vi "Read.vi"(8 "error in":errorcluster, 11 "TPCANHandle in":T2=81 items=["PCAN_NONEBUS"=0, "PCAN_USBBUS1"=81, "PCAN_USBBUS2"=82, "PCAN_USBBUS3"=83, "PCAN_USBBUS4"=84, "PCAN_USBBUS5"=85, "PCAN_USBBUS6"=86, "PCAN_USBBUS7"=87, "PCAN_USBBUS8"=88, "PCAN_USBBUS9"=1289, "PCAN_USBBUS10"=1290, "PCAN_USBBUS11"=1291, "PCAN_USBBUS12"=1292, "PCAN_USBBUS13"=1293, "PCAN_USBBUS14"=1294, "PCAN_USBBUS15"=1295, "PCAN_USBBUS16"=1296]) -> (0 "error out":errorcluster, 1 "Time Stamp":timestamp format="%<%x %.3X>T", 2 "PCAN Message":T3 {"DATA"."7" format="%.0x"; "DATA"."6" format="%.0x"; "DATA"."5" format="%.0x"; "DATA"."4" format="%.0x"; "DATA"."3" format="%.0x"; "DATA"."2" format="%.0x"; "DATA"."1" format="%.0x"; "DATA"."0" format="%.0x"; "MSGTYPE" items=["STANDARD"=0, "RTR"=1, "EXTENDED"=2, "FD"=4, "BRS"=8, "ESI"=16, "ECHO"=32, "ERRFRAME"=64, "STATUS"=128]}, 3 "TPCANHandle out":T2=81 items=["PCAN_NONEBUS"=0, "PCAN_USBBUS1"=81, "PCAN_USBBUS2"=82, "PCAN_USBBUS3"=83, "PCAN_USBBUS4"=84, "PCAN_USBBUS5"=85, "PCAN_USBBUS6"=86, "PCAN_USBBUS7"=87, "PCAN_USBBUS8"=88, "PCAN_USBBUS9"=1289, "PCAN_USBBUS10"=1290, "PCAN_USBBUS11"=1291, "PCAN_USBBUS12"=1292, "PCAN_USBBUS13"=1293, "PCAN_USBBUS14"=1294, "PCAN_USBBUS15"=1295, "PCAN_USBBUS16"=1296], 4 "Receive Queue empty":bool, 5 "TPCANStatus":T1 items=["PCAN_ERROR_OK"=0, "PCAN_ERROR_XMTFULL"=1, "PCAN_ERROR_OVERRUN"=2, "PCAN_ERROR_BUSLIGHT"=4, "PCAN_ERROR_BUSHEAVY"=8, "PCAN_ERROR_BUSPASSIVE"=262144, "PCAN_ERROR_BUSOFF"=16, "PCAN_ERROR_QRCVEMPTY"=32, "PCAN_ERROR_QOVERRUN"=64, "PCAN_ERROR_QXMTFULL"=128, "PCAN_ERROR_REGTEST"=256, "PCAN_ERROR_NODRIVER"=512, "PCAN_ERROR_HWINUSE"=1024, "PCAN_ERROR_NETINUSE"=2048, "PCAN_ERROR_ILLHW"=5120, "PCAN_ERROR_ILLNET"=6144, "PCAN_ERROR_ILLCLIENT"=7168, "PCAN_ERROR_RESOURCE"=8192, "PCAN_ERROR_ILLPARAMTYPE"=16384, "PCAN_ERROR_ILLPARAMVAL"=32768, "PCAN_ERROR_UNKNOWN"=65536, "PCAN_ERROR_ILLDATA"=131072, "PCAN_ERROR_ILLMODE"=524288, "PCAN_ERROR_CAUTION"=33554432, "PCAN_ERROR_INITIALIZE"=67108864, "PCAN_ERROR_ILLOPERATION"=134217728])   [LabVIEW 2018, in "PCANBasic.lvlib"]
doc: "Reads a CAN message and its time stamp from the receive queue of a PCAN Channel.\n\nTimestamps on Linux are the number of milliseconds that have elapsed since the epoch: the epoch is the point in time of 00:00 UTC, 1 January 1970.\n\nThe Read method returns received messages or status messages from the receive queue. It is important to call Read repeatedly until the queue is empty. In case there are no more messages in queue, the value PCAN_ERROR_QRCVEMPTY is returned. The error code PCAN_ERROR_QRCVEMPTY is also returned if the reception of messages is disabled. See Receive Status Parameter for more information. \n\nThe receive queue can contain up to 32767 messages. \n\nIf the time when the message was received is not needed, use the overloaded Read method. \n\nThere are two possibilities for reading messages from the receive queue of a Channel: \n\nTime-Triggered Reading: Consists in periodically calls to the Read method. Typically, an application starts a timer that every 50 or 100 milliseconds check for messages, calling the Read method in a loop until the value of PCAN_ERROR_QRCVEMTY or another error condition is reached. \n\nEvent-Triggered Reading: Consists in reacting to a notification sent by the PCAN driver to a registered application, when a message is received and inserted in its receive queue. See Using Events to obtain more information about reading with events. \n\nAbout bus errors / Status messages \n\nIf a bus-off error occurs, an application cannot use the channel to communicate anymore, until the CAN controller is reset. With PCAN-Basic it is not possible to reset the CAN controller through a method directly. Consider using the PCAN-Basic property PCAN_BUSOFF_AUTORESET which instructs the API to reset the CAN controller when a bus-off state is detected automatically. \n\nAnother ways to reset errors like bus-off, bus-heavy and bus-light:\n\nPerforming an uninitialize / initialize cycle: This causes a hardware reset, but only when no more clients are connected to that channel. \nUsing the parameter PCAN_HARD_RESET_STATUS: It instructs this method to explicitly perform a hardware reset regardless of whether other clients are connected to that channel. \nThe message type (see TPCANMessageType) of a CAN message indicates if the message is a 11-bit, 29-bit, RTR, Error, or Status message. This value should be checked every time a message has been read successfully. \n\nIf the bit PCAN_MESSAGE_ERRFRAME is set in the TPCANMsg.MSGTYPE field, the message is an Error frame (see Error Frames). \n\nIf the bit PCAN_MESSAGE_STATUS is set in the TPCANMsg.MSGTYPE field, the message is a Status message. The ID and LEN fields do not contain valid data. The first 4 data bytes of the message contain the Error Code. The MSB of the Error Code is in data byte 0, the LSB is in data byte 3."
uses:
  PCANBasic.lvlib
  PCAN Message types.ctl
  PCAN Message.ctl
  PCAN Timestamp.ctl
  TPCANHandle.ctl
  TPCANStatus.ctl
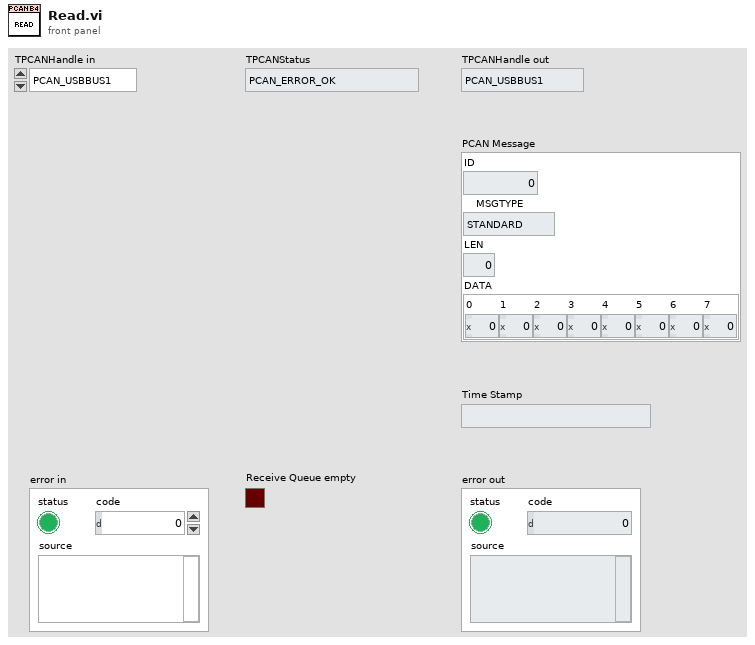
[diagram p1: front panel]
types:
  T1 = typedef "PCANBasic.lvlib/TPCANStatus.ctl" = u32
  T2 = typedef "PCANBasic.lvlib/TPCANHandle.ctl" = u16
  T3 = typedef "PCANBasic.lvlib/PCAN Message.ctl" = cluster{"ID":u32, "MSGTYPE":T4, "LEN":u8, "DATA":cluster{"0":u8, "1":u8, "2":u8, "3":u8, "4":u8, "5":u8, "6":u8, "7":u8}}
  T4 = typedef "PCANBasic.lvlib/PCAN Message types.ctl" = u8
  T5 = typedef "PCANBasic.lvlib/PCAN Timestamp.ctl" = cluster{"millis":u32, "millis overflow":u16, "micros":u16}
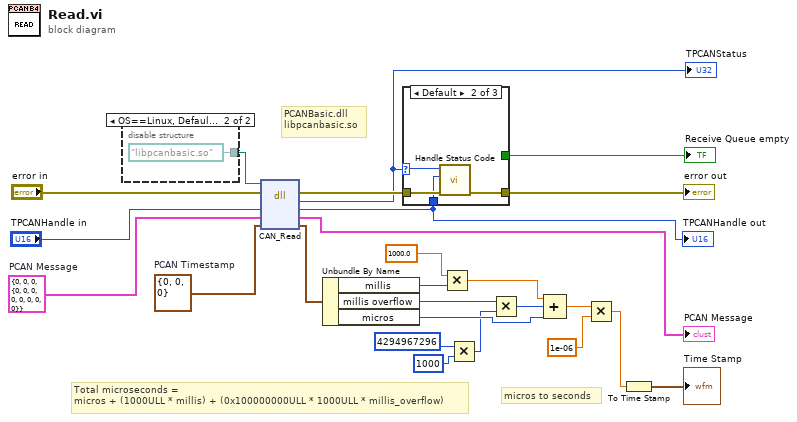
[diagram p0: block diagram]
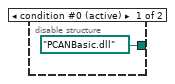
[diagram p2: hidden frame]
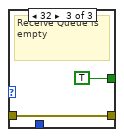
[diagram p4: hidden frame]
diagram:
  w23 = T5 {"millis"=0, "millis overflow"=0, "micros"=0}  # PCAN Timestamp
  w24 = T3 {"ID"=0, "MSGTYPE"=0, "LEN"=0, "DATA"={"0"=0, "1"=0, "2"=0, "3"=0, "4"=0, "5"=0, "6"=0, "7"=0}}  # PCAN Message
  # "PCANBasic.dll\nlibpcanbasic.so"
  # "micros to seconds"
  # "Total microseconds = \nmicros + (1000ULL * millis) + (0x100000000ULL * 1000ULL * millis_overflow)"
  n1 = disable-structure shown="OS==Linux, Default" {
    disable-tunnel: [path "PCANBasic.dll" path "libpcanbasic.so"] -> w4
    frame condition #0 (active) {
    }
    frame condition #1 {
    }
  }
  n2 = dll-call lib="?" fn="CAN_Read"(path in=w4, error in="error in", "Channel"="TPCANHandle in", "MessageBuffer"=w24, "TimestampBuffer"=w23) -> (error out=w12:errorcluster, "TPCANStatus"=w2:u32, "Channel"=w1:u16, "MessageBuffer"=→"PCAN Message":T3, "TimestampBuffer"=w21:T5)  [unwired: 1 in, 1 out]
  "TPCANHandle out" <- w1
  "TPCANStatus" <- w2
  n3 = Unbundle By Name(w21) -> ("millis"=w20:u32, "millis overflow"=w17:u16, "micros"=w18:u16)
  n4 = case shown="Default" w2 {
    selector: w2 -> [_ w30 _]
    tunnel: w12 -> [w28 w32 w34]
    tunnel: [w28 w31 w34] -> w11
    tunnel: [_ _ TRUE] -> w5
    tunnel: w1 -> [_ w29 _]
    frame 0 {
    }
    frame Default {
      n5 = call "Handle Status Code.vi"("error in"=w32, "TPCANHandle"=w29, "TPCANStatus"=w30) -> ("error out"=w31:errorcluster)  [unwired: 8 in]
    }
    frame 32 {
      # "Receive Queue is empty"
    }
  }
  "error out" <- w11
  "Receive Queue empty" <- w5
  n6 = Multiply(x=1000.0, y=w20) -> (x*y=w15:dbl)
  n7 = Multiply(x=u64 4294967296, y=u64 1000) -> (x*y=w6:u64)
  n8 = Multiply(x=w17, y=w6) -> (x*y=w16:u64)
  n9 = Compound Arithmetic op=ADD(w15, w16, w18) -> (w14:dbl)
  n10 = Multiply(x=w14, y=1e-06) -> (x*y=w10:dbl)
  n11 = To Time Stamp(1:w10) -> (0:→"Time Stamp":timestamp)
